vi "CMI Sync V3 Open.vi"(8 "error in":errorcluster, 11 "session in":T1={"VISA"="", "baud rate [bd/s]"=115200, "source"=enum."Auto", "hv range"=enum."1kV", "fsrc is fixed"=FALSE, "fsrc [Hz]"=10000000.0, "freq integ [s]"=1.0, "freq filter"=5, "trig level"=enum."TTL 5V", "chn1 mode"=enum."Source divider", "chn1 level"=enum."Positive 5V", "chn2 mode"=enum."Source divider", "chn2 level"=enum."Positive 5V", "chn2 div"=1, "chn3 mode"=enum."Chn 1 Active", "chn3 level"=enum."Positive 5V", "chn1 div entry"=enum."Calculate nearest divisor from measured fx", "chn1 dev limit [%]"=1.0, "chn1 check dev"=FALSE} {"chn2 div" min=1 max=100000000 step=1; "fsrc [Hz]" format="%_8p"}) -> (0 "error out":errorcluster, 2 "identification string":string, 3 "session out":T1={"VISA"="", "baud rate [bd/s]"=115200, "source"=enum."Auto", "hv range"=enum."1kV", "fsrc is fixed"=FALSE, "fsrc [Hz]"=10000000.0, "freq integ [s]"=1.0, "freq filter"=5, "trig level"=enum."TTL 5V", "chn1 mode"=enum."Source divider", "chn1 level"=enum."Positive 5V", "chn2 mode"=enum."Source divider", "chn2 level"=enum."Positive 5V", "chn2 div"=1, "chn3 mode"=enum."Chn 1 Active", "chn3 level"=enum."Positive 5V", "chn1 div entry"=enum."Calculate nearest divisor from measured fx", "chn1 dev limit [%]"=1.0, "chn1 check dev"=FALSE} {"chn2 div" min=1 max=100000000 step=1; "fsrc [Hz]" format="%_8p"})   [LabVIEW 2020, in "AWG.lvlib" / "CMI Sync Unit V3.lvlib"]
doc: "Initializes sync unit with defaul baud rate."
uses:
  CMI Sync Unit V3.lvlib
  CMI Sync V3 session.ctl
  Configure/CMI Sync V3 Reference Clock Source.ctl
  Configure/CMI Sync V3 HV input Range.ctl
  Configure/CMI Sync V3 Trigger Input Level.ctl
  Configure/CMI Sync V3 Channel 1 Mode.ctl
  Configure/CMI Sync V3 Channel Output Levels.ctl
  Configure/CMI Sync V3 Channel 2 Mode.ctl
  Configure/CMI Sync V3 Channel 3 Mode.ctl
  Configure/CMI Sync V3 Channel 1 Divisor Entry Mode.ctl
  <vilib>/Utility/error.llb/Error Cluster From Error Code.vi
  <vilib>/ErrorRing/Error Ring.xnode
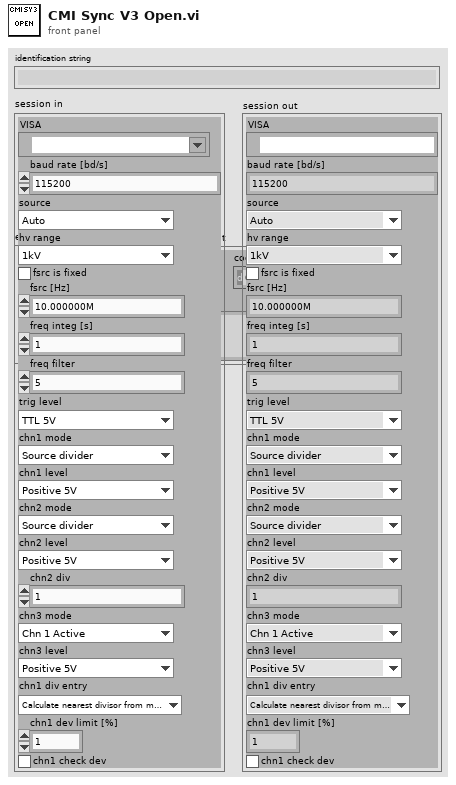
[diagram p1: front panel]
types:
  T1 = typedef "AWG.lvlib/CMI Sync Unit V3.lvlib/CMI Sync V3 session.ctl" = cluster{"VISA":refnum<visa-resource-name>, "baud rate [bd/s]":i32, "source":T2, "hv range":T3, "fsrc is fixed":bool, "fsrc [Hz]":dbl, "freq integ [s]":dbl, "freq filter":i32, "trig level":T4, "chn1 mode":T5, "chn1 level":T6, "chn2 mode":T7, "chn2 level":T6, "chn2 div":i32, "chn3 mode":T8, "chn3 level":T6, "chn1 div entry":T9, "chn1 dev limit [%]":dbl, "chn1 check dev":bool}
  T2 = typedef "AWG.lvlib/CMI Sync Unit V3.lvlib/CMI Sync V3 Reference Clock Source.ctl" = enum16{"Auto", "Internal", "Logic", "Sine", "HV"}
  T3 = typedef "AWG.lvlib/CMI Sync Unit V3.lvlib/CMI Sync V3 HV input Range.ctl" = enum16{"10V", "60V", "250V", "1kV"}
  T4 = typedef "AWG.lvlib/CMI Sync Unit V3.lvlib/CMI Sync V3 Trigger Input Level.ctl" = enum16{"LVCMOS 3V3", "TTL 5V"}
  T5 = typedef "AWG.lvlib/CMI Sync Unit V3.lvlib/CMI Sync V3 Channel 1 Mode.ctl" = enum16{"Source divider", "DDS absolute", "DDS ratio", "DDS ratio M/N"}
  T6 = typedef "AWG.lvlib/CMI Sync Unit V3.lvlib/CMI Sync V3 Channel Output Levels.ctl" = enum16{"Positive 3V3", "Negative 3V3", "Positive 5V", "Negative 5V"}
  T7 = typedef "AWG.lvlib/CMI Sync Unit V3.lvlib/CMI Sync V3 Channel 2 Mode.ctl" = enum16{"Source divider", "Chn 1 divide"}
  T8 = typedef "AWG.lvlib/CMI Sync Unit V3.lvlib/CMI Sync V3 Channel 3 Mode.ctl" = enum16{"Chn 1 Active", "Chn 2 Active", "Chn 1 Trigger", "Chn 2 Trigger", "Gate", "PPS", "10MHz"}
  T9 = typedef "AWG.lvlib/CMI Sync Unit V3.lvlib/CMI Sync V3 Channel 1 Divisor Entry Mode.ctl" = enum16{"Set divisor directly", "Calculate nearest divisor from measured fx"}
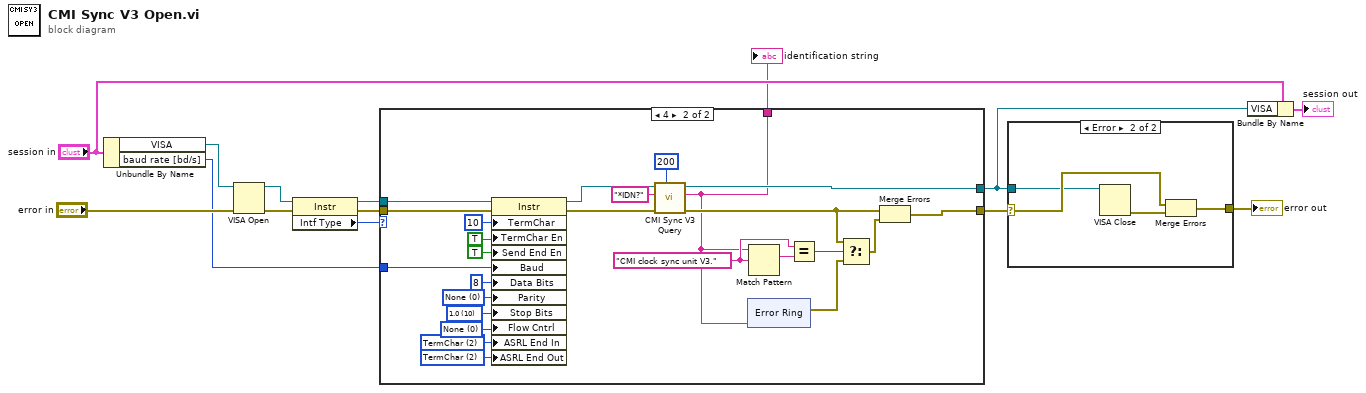
[diagram p0: block diagram]
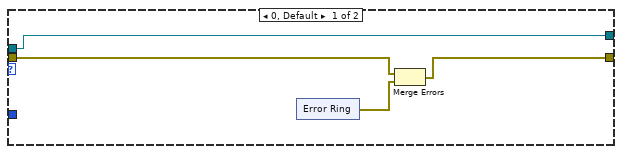
[diagram p3: hidden frame]
diagram:
  n1 = Unbundle By Name("session in") -> ("VISA"=w13:refnum<visa-resource-name>, "baud rate [bd/s]"=w7:i32)
  n2 = VISA Open(error in (no error)="error in", VISA resource name=w13) -> (VISA resource name=w11:refnum<visa-resource-name>, error out=w12:errorcluster)  [unwired: 3 in]
  n3 = property class="Instr"(reference=w11, error in=w12) -> (reference out=w9:refnum<visa-resource-name>, error out=w8:errorcluster, "Intf Type"=w10:u16)
  n4 = case shown="4" w10 {
    tunnel: w9 -> [w18 w37]
    tunnel: w8 -> [w16 w38]
    tunnel: w7 -> [_ w48]
    tunnel: [w15 w26] -> w6
    tunnel: [w18 w25] -> w3
    tunnel: [_ w24] -> w1
    frame 0, Default {
      n5 = xnode "Error Ring"() -> ("error out"=w17:errorcluster)
      n6 = Merge Errors(w16, w17) -> (w15:errorcluster)
    }
    frame 4 {
      w31 = "CMI clock sync unit V3." ("regular expression")
      w42 = u16 2 items=["None", "Last Bit", "TermChar", "Break"] ("Serial Settings:End Mode for Writes")
      w43 = u16 2 items=["None", "Last Bit", "TermChar"] ("Serial Settings:End Mode for Reads")
      w44 = u16 0 items=["None", "XON/XOFF", "RTS/CTS", "XON/XOFF & RTS/CTS", "DTR/DSR", "XON/XOFF & DTR/DSR"] ("Serial Settings:Flow Control")
      w45 = u16 10 items=["1.0"=10, "1.5"=15, "2.0"=20] ("Serial Settings:Stop Bits")
      w46 = u16 0 items=["None", "Odd", "Even", "Mark", "Space"] ("Serial Settings:Parity")
      n7 = property class="Instr"(reference=w37, error in=w38, "TermChar"=u8 10 ("Message Based Settings:Termination Character"), "TermChar En"=TRUE ("Message Based Settings:Termination Character Enable"), "Send End En"=TRUE ("Message Based Settings:Send End Enable"), "Baud"=w48, "Data Bits"=u16 8 ("Serial Settings:Data Bits"), "Parity"=w46, "Stop Bits"=w45, "Flow Cntrl"=w44, "ASRL End In"=w43, "ASRL End Out"=w42) -> (reference out=w35:refnum<visa-resource-name>, error out=w36:errorcluster)
      n8 = call "CMI Sync V3 Query.vi"("read byte count (100)"=u32 200, "error in"=w36, "command"="*IDN?" ("write buffer"), "VISA in"=w35) -> ("error out"=w28:errorcluster, "read buffer"=w24:string, "VISA resource name out"=w25:refnum<visa-resource-name>)  [unwired: 5 in]
      n9 = xnode "Error Ring"("parameter 0"=w24) -> ("error out"=w29:errorcluster)
      n10 = Match Pattern(string=w24, regular expression=w31) -> (match substring=w32:string)  [unwired: 1 in, 3 out]
      n11 = Equal?(x=w31, y=w32) -> (x = y?=w30:bool)
      n12 = Select(t=w28, s=w30, f=w29) -> (s? t:f=w27:errorcluster)
      n13 = Merge Errors(w28, w27) -> (w26:errorcluster)
    }
  }
  "identification string" <- w1
  n14 = case shown="Error" w6 {
    selector: w6 -> [w56 w59]
    tunnel: [w56 w58] -> w5
    tunnel: w3 -> [_ w57]
    frame No Error {
    }
    frame Error {
      n15 = VISA Close(VISA resource name=w57) -> (error out=w60:errorcluster)  [unwired: 1 in]
      n16 = Merge Errors(w59, w60) -> (w58:errorcluster)
    }
  }
  "error out" <- w5
  n17 = Bundle By Name(cluster="session in", "VISA"=w3) -> (→"session out":T1)
